vi "_DebugV1.0+IVcurve.vi"() -> ()   [LabVIEW 2017]
uses:
  <vilib>/Instr/_visa.llb/VISA Configure Serial Port (Instr).vi
  <vilib>/Analysis/NI_AALPro.lvlib
panel:
  out "Vres/Vin, %":dbl
  out "Vres":cluster{dbl[], dbl[]}(graph)
  out "PlotPoints":cluster{"Time":dbl[], "Voltage":dbl[]}(graph)={"Time"=[0.0, 0.00037111111108161925, 0.000510833333311085, 0.0006505555555405509, 0.0007766666666915019, 0.0009172222221968695, 0.0010569444444263353, 0.0011958333333152243, 0.0013350000000274223], "Voltage"=[5.89, 5.89, 5.89, 5.89, 5.89, 5.89, 5.89, 5.89, 5.89]}
  out "IV curve":cluster{dbl[], dbl[]}(graph)
  out "VoltageRes, V":dbl
  in  "film H, nm":dbl=50.0
  in  "6 electrodes":bool
  out "Numeric":i32
  out "Current":cluster{dbl[], dbl[]}(graph)
  out "DAC1volt, V":dbl
  out "Bytes at Port":u32
  out "RecTry":i32
  out "OutVoltage, V":dbl
  out "Knob":u32
  out "Current, mA":dbl format="%#_4g"
  out "Channel 1, V":dbl format="%#_5g"
  in  "Stop Button":bool
  in  "Start Button":bool
  out "VoltageArray, V":dbl[](array[numeric])
  in  "Step, V":dbl=1.0
  in  "Amplitude, V":dbl=1.0
  in  "LOG file":path
  in  "COM port":refnum<visa-resource-name>
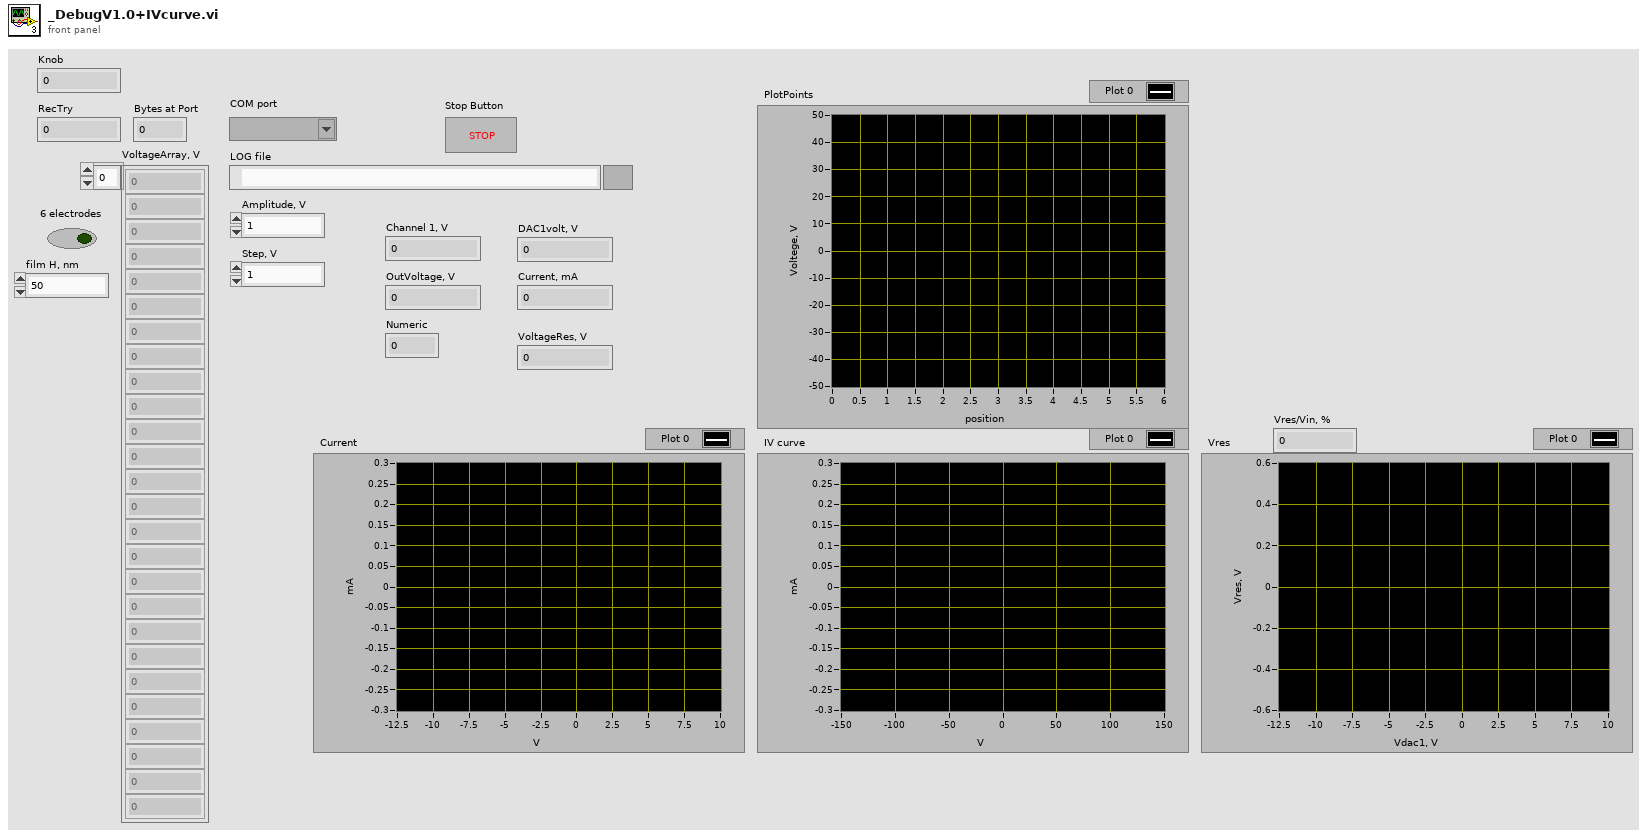
[diagram p1: front panel]
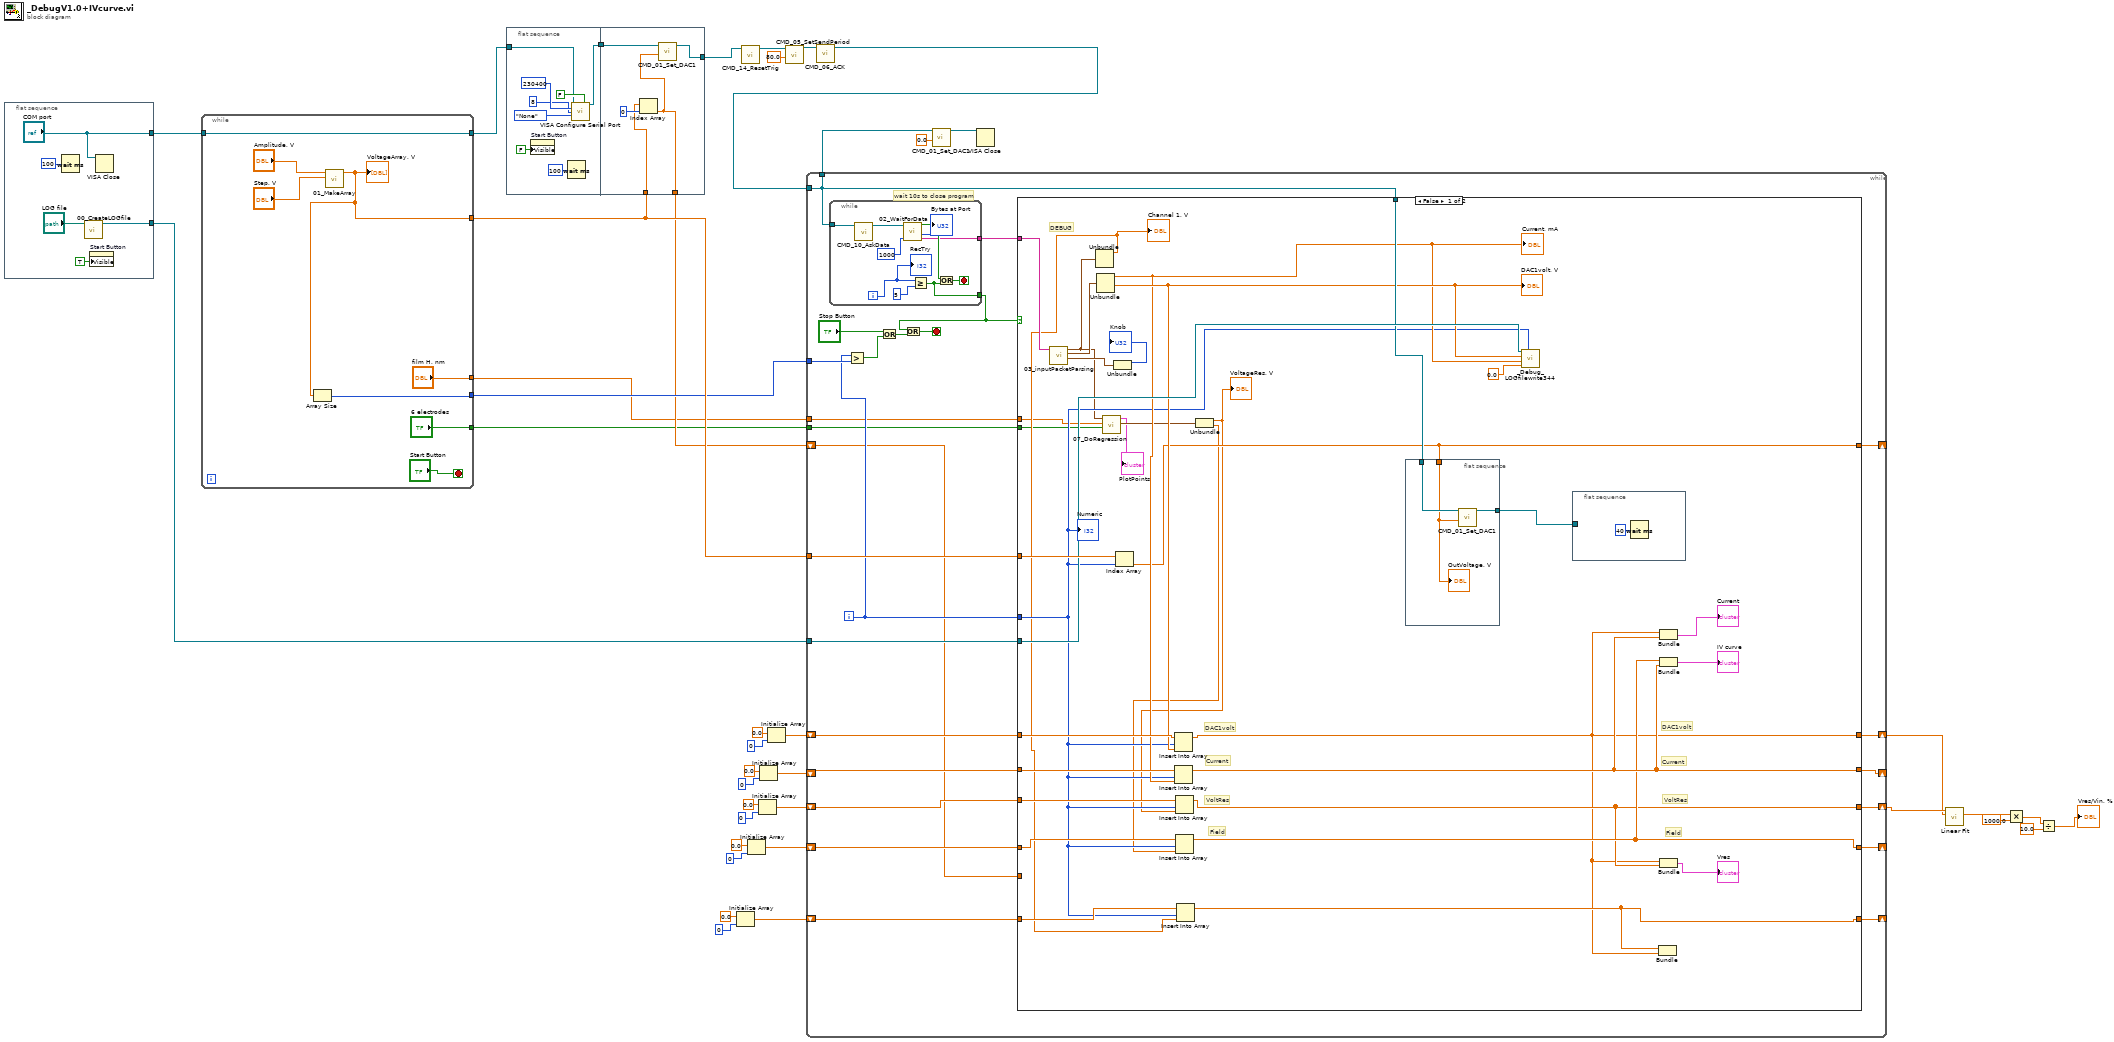
[diagram p0: block diagram]
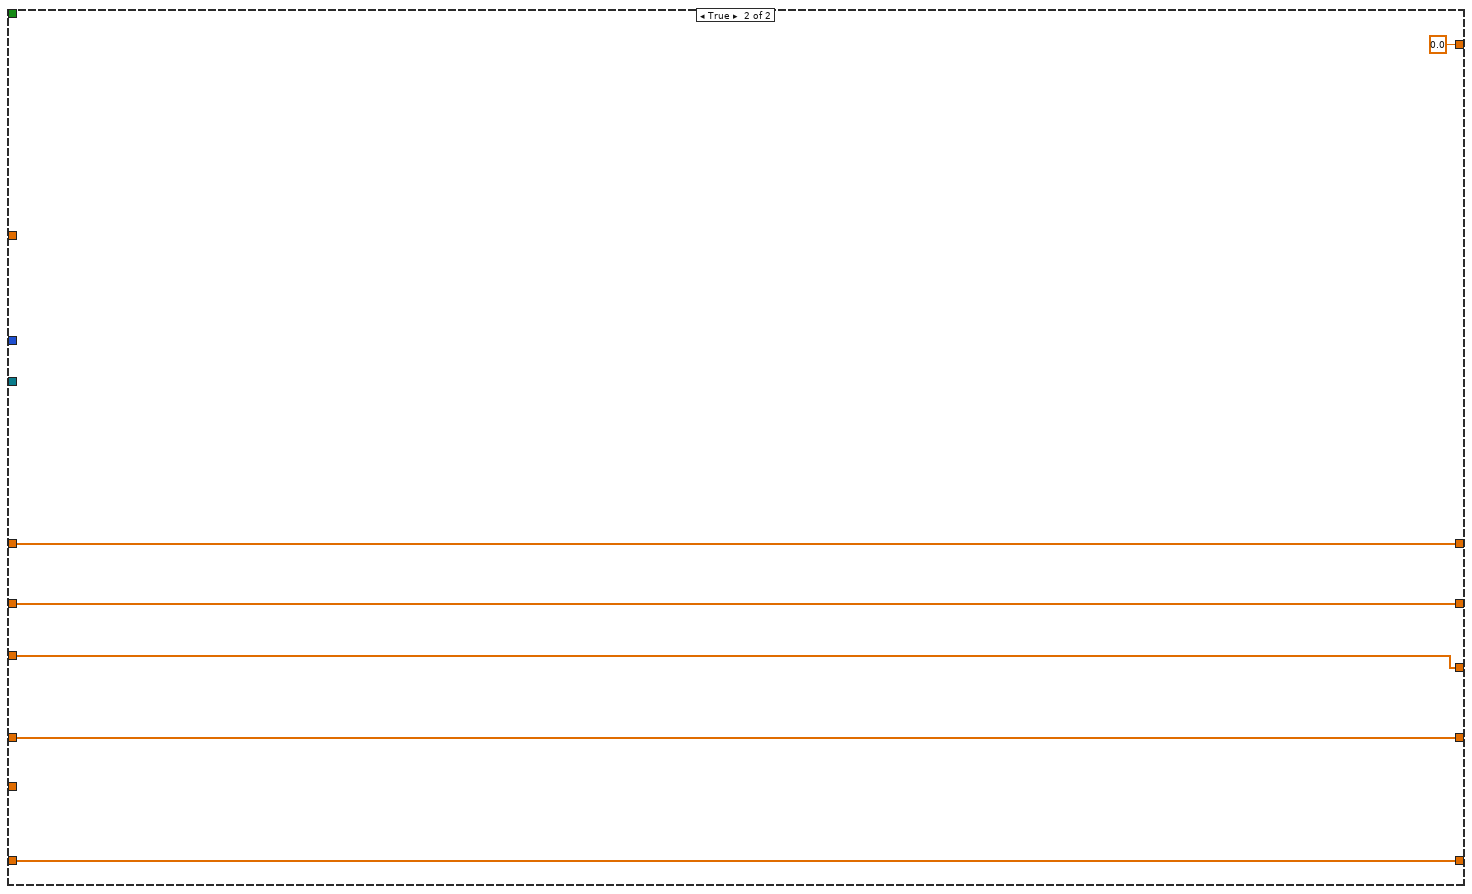
[diagram p2: hidden frame]
diagram:
  n1 = flat-sequence {
    tunnel: ["COM port"] -> w39
    tunnel: [w41] -> w37
    frame #0 {
      n2 = Wait (ms)(milliseconds to wait=u32 100) -> ()  [unwired: 1 out]
      n3 = call "00_CreateLOGfile.vi"("LOG file"="LOG file") -> ("refnum out"=w41:refnum<file>)  [unwired: 10 in]
      n4 = property on="Start Button" class="Bool"("Visible"=TRUE) -> ()  [unwired: 2 in, 2 out]
      n5 = VISA Close(VISA resource name="COM port") -> ()  [unwired: 1 in, 1 out]
    }
  }
  n6 = while {
    tunnel: w39 -> [w49]
    tunnel: [w49] -> w38
    tunnel: [w48] -> w27
    tunnel: [w47] -> w26
    tunnel: ["6 electrodes"] -> w9
    tunnel: ["film H, nm"] -> w8
    stop <- "Start Button" stop-if-true
    n7 = call "01_MakeArray.vi"("Amp"="Amplitude, V", "Step"="Step, V") -> ("Array"=w48:dbl[])  [unwired: 8 in]
    "VoltageArray, V" <- w48
    n8 = Array Size(array=w48) -> (size(s)=w47:i32)
  }
  n9 = flat-sequence {
    tunnel: w38 -> [w56]
    tunnel: [w55] -> w28
    tunnel: [w64] -> w35
    tunnel: w28 -> [w63]
    tunnel: w27 -> [w62]
    tunnel: [w61] -> w13
    frame #0 {
      n10 = property on="Start Button" class="Bool"("Visible"=FALSE) -> ()  [unwired: 2 in, 2 out]
      n11 = Wait (ms)(milliseconds to wait=u32 100) -> ()  [unwired: 1 out]
      n12 = call-poly "VISA Configure Serial Port"("VISA resource name"=w56, "Enable Termination\nChar (T)"=FALSE ("Enable Termination\nChar (T)"), "baud rate (9600)"=u32 230400, "data bits (8)"=u16 8, "parity (0:none)"=enum16{"None", "Odd", "Even", "Mark", "Space"}."None") -> ("VISA resource name out"=w55:refnum<visa-resource-name>)  [unwired: 9 in, 1 out]
    }
    frame #1 {
      n13 = Index Array(array=w62, index=0) -> (element=w61:dbl)
      n14 = call "CMD_01_Set_DAC1.vi"("Input, V"=w61, "VISA resource name"=w63) -> ("VISA resource name out"=w64:refnum<visa-resource-name>)  [unwired: 9 in]
    }
  }
  n15 = Initialize Array(0.0 ("element"), 0 ("dimension size")) -> (w10:dbl[])
  n16 = call "CMD_14_ResetTrig.vi"("VISA resource name"=w35) -> ("VISA resource name out"=w31:refnum<visa-resource-name>)  [unwired: 10 in]
  n17 = Initialize Array(0.0 ("element"), 0 ("dimension size")) -> (w14:dbl[])
  n18 = Initialize Array(0.0 ("element"), 0 ("dimension size")) -> (w17:dbl[])
  n19 = Initialize Array(0.0 ("element"), 0 ("dimension size")) -> (w20:dbl[])
  n20 = Initialize Array(0.0 ("element"), 0 ("dimension size")) -> (w25:dbl[])
  n21 = call "CMD_05_SetSendPeriod.vi"("Period, ms"=80.0, "VISA resource name"=w31) -> ("VISA resource name out"=w30:refnum<visa-resource-name>)  [unwired: 9 in]
  n22 = call "CMD_06_ACK.vi"("VISA resource name"=w30) -> ("VISA resource name out"=w29:refnum<visa-resource-name>)  [unwired: 10 in]
  n23 = while {
    tunnel: w29 -> [w85]
    tunnel: [w85] -> w36
    tunnel: w27 -> [w86]
    tunnel: w37 -> [w87]
    tunnel: w26 -> [w82]
    shift-right: [w76] -> w1
    shift-left: w25 -> [w77]
    shift-right: [w75] -> _
    shift-left: w20 -> [w78]
    shift-right: [w74] -> w2
    shift-left: w17 -> [w79]
    shift-right: [w72] -> _
    shift-left: w14 -> [w73]
    shift-right: [w71] -> _
    shift-left: w13 -> [w70]
    shift-right: [w68] -> _
    shift-left: w10 -> [w69]
    tunnel: w9 -> [w67]
    tunnel: w8 -> [w66]
    i -> [w80]
    stop <- w90 stop-if-true
    # "wait 10s to close program"
    n24 = while {
      tunnel: w85 -> [w136]
      tunnel: [w139] -> w89
      tunnel: [w140] -> w88
      i -> [w138]
      stop <- w142 stop-if-true
      n25 = call "CMD_10_AskData.vi"("VISA resource name"=w136) -> ("VISA resource name out"=w135:refnum<visa-resource-name>)  [unwired: 10 in]
      n26 = call "02_WaitForData.vi"("WaitTimeoutMS"=u32 1000, "VISA"=w135) -> ("Buffer"=w140:string, "Bytes at Port"=→"Bytes at Port":u32, "Data Recived"=w141:bool)  [unwired: 7 in]
      n27 = Greater Or Equal?(x=w138, y=5) -> (x >= y?=w139:bool)
      n28 = Or(x=w141, y=w139) -> (x .or. y?=w142:bool)
      "RecTry" <- w138
    }
    n29 = Greater?(x=w80, y=w82) -> (0:w81:bool)
    n30 = Or(x="Stop Button", y=w81) -> (x .or. y?=w84:bool)
    n31 = Or(x=w89, y=w84) -> (x .or. y?=w90:bool)
    n32 = case shown="False" w89 {
      tunnel: w88 -> [w119 _]
      tunnel: w87 -> [w120 _]
      tunnel: w80 -> [w107 _]
      tunnel: w86 -> [w121 _]
      tunnel: w85 -> [w118 _]
      tunnel: w79 -> [w117 w132]
      tunnel: w78 -> [w116 w133]
      tunnel: w77 -> [w115 w134]
      tunnel: [w91 w134] -> w76
      tunnel: [w98 w133] -> w75
      tunnel: [w92 w132] -> w74
      tunnel: w73 -> [w111 w131]
      tunnel: [w95 w131] -> w72
      tunnel: [w110 0.0] -> w71
      tunnel: w70 -> [_ _]
      tunnel: w69 -> [w108 w129]
      tunnel: [w93 w129] -> w68
      tunnel: w67 -> [w103 _]
      tunnel: w66 -> [w102 _]
      frame False {
        # "Field"
        # "Field"
        # "VoltRes"
        # "DAC1volt"
        # "Current"
        # "VoltRes"
        # "DAC1volt"
        # "Current"
        # "DEBUG"
        n33 = call "03_inputPacketParsing.vi"("string"=w119) -> ("Service state"=w122:cluster{u8, u8}, "DAC state"=w124:cluster{dbl, dbl, dbl, dbl}, "Voltage"=w104:cluster{dbl, dbl, dbl, dbl})  [unwired: 6 in, 2 out]
        n34 = Unbundle(w104) -> (w106:dbl)  [unwired: 3 out]
        "Channel 1, V" <- w106
        n35 = Unbundle(w124) -> (w113:dbl, w114:dbl)  [unwired: 2 out]
        "Current, mA" <- w113
        "DAC1volt, V" <- w114
        n36 = call "07_DoRegression.vi"("6 electrodes"=w103, "film H, nm"=w102, "Input ChVoltage"=w104) -> ("Regression"=w101:cluster{"VoltageRes, V":dbl, "Field, kV/cm":dbl}, "PlotPoints"=→"PlotPoints":cluster{"Time":dbl[], "Voltage":dbl[]})  [unwired: 6 in, 1 out]
        n37 = Unbundle(w122) -> (→"Knob":u8)  [unwired: 1 out]
        n38 = Index Array(array=w121, index=w107) -> (element=w110:dbl)
        n39 = Insert Into Array(array=w115, index=w107, new element=w114) -> (w91:dbl[])
        n40 = Insert Into Array(array=w116, index=w107, new element=w113) -> (w98:dbl[])
        n41 = Insert Into Array(array=w108, index=w107, new element=w106) -> (w93:dbl[])
        n42 = Unbundle(w101) -> ("VoltageRes, V"=w100:dbl, "Field, kV/cm"=w96:dbl)
        "VoltageRes, V" <- w100
        n43 = Insert Into Array(array=w117, index=w107, new element=w100) -> (w92:dbl[])
        n44 = Insert Into Array(array=w111, index=w107, new element=w96) -> (w95:dbl[])
        n45 = flat-sequence {
          tunnel: w110 -> [w126]
          tunnel: w118 -> [w128]
          tunnel: [w127] -> w109
          frame #0 {
            n46 = call "CMD_01_Set_DAC1.vi"("Input, V"=w126, "VISA resource name"=w128) -> ("VISA resource name out"=w127:refnum<visa-resource-name>)  [unwired: 9 in]
            "OutVoltage, V" <- w126
          }
        }
        n47 = call "_Debug_LOGfilewrite344.vi"("N"=w107, "344cur"=0.0, "DAC1cur"=w113, "DAC1volt2"=w114, "refnum out"=w120) -> ()  [unwired: 7 in]
        n48 = flat-sequence {
          tunnel: w109 -> [_]
          frame #0 {
            n49 = Wait (ms)(milliseconds to wait=u32 40) -> ()  [unwired: 1 out]
          }
        }
        n50 = Bundle(w93, w91) -> ()  [unwired: 1 in, 1 out]
        n51 = Bundle(w91, w98) -> (→"Current":cluster{dbl[], dbl[]})  [unwired: 1 in]
        n52 = Bundle(w95, w98) -> (→"IV curve":cluster{dbl[], dbl[]})  [unwired: 1 in]
        n53 = Bundle(w91, w92) -> (→"Vres":cluster{dbl[], dbl[]})  [unwired: 1 in]
        "Numeric" <- w107
      }
      frame True {
      }
    }
  }
  n54 = call "CMD_01_Set_DAC1.vi"("Input, V"=0.0, "VISA resource name"=w36) -> ("VISA resource name out"=w33:refnum<visa-resource-name>)  [unwired: 9 in]
  n55 = VISA Close(VISA resource name=w33) -> ()  [unwired: 1 in, 1 out]
  n56 = call <vilib>:"Linear Fit.vi"("Y"=w2, "X"=w1) -> ("slope"=w7:dbl)  [unwired: 9 in, 4 out]
  n57 = Multiply(x=w7, y=1000.0) -> (x*y=w4:dbl)
  n58 = Divide(x=w4, y=10.0) -> (x/y=→"Vres/Vin, %":dbl)
